vi "ECT verification.vi"(0 ".NET Refnum in":refnum<k24>, 5 "Cal ECT (sec)":u16, 7 "Time remaining (sec)":u16, 11 "error in":errorcluster) -> (3 "Expected SSD":string, 4 ".NET Refnum out":refnum<k24>, 6 "Expected ECT (sec)":u16, 8 "Actual ECT (sec)":u16, 10 "ECT Pass/Fail":bool, 14 "Report Text":string, 15 "error out":errorcluster)   [LabVIEW 2016, in "TL27.lvlib"]
uses:
  Projects/TL27.lvlib
  C:/Automation/DLLs/PC Dot Net/GeaCommunication.dll
  Common/LabVIEW GEA2 Toolkit/LabVIEW_GEA2_Toolkit.lvlibp/type defs/Source_Destination.ctl
  Common/LabVIEW GEA2 Toolkit/LabVIEW_GEA2_Toolkit.lvlibp/type defs/ERD Read Data In.ctl
  Common/LabVIEW GEA2 Toolkit/LabVIEW_GEA2_Toolkit.lvlibp/type defs/Data Type.ctl
  Valew Common/Display/controls/HEUI_Display_Care.ctl
  Valew Common/Display/controls/HEUI_Display.ctl
  Valew Common/Display/controls/Cycle Selection Enum.ctl
  Valew Common/Display/controls/Stain Enum.ctl
  Valew Common/Display/controls/Temp Enum.ctl
  Valew Common/Display/controls/Soil Enum.ctl
  Valew Common/Display/controls/Spin Enum.ctl
  Valew Common/Display/controls/750 Status Enum.ctl
  Common/LabVIEW GEA2 Toolkit/LabVIEW_GEA2_Toolkit.lvlibp
panel:
  out "Diffrence":i16
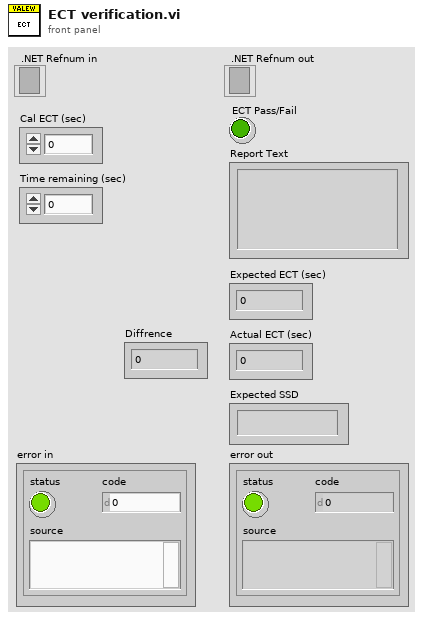
[diagram p1: front panel]
types:
  T1 = typedef "LabVIEW_GEA2_Toolkit.lvlibp/Source_Destination.ctl" = cluster{"Source":u8, "Destination":u8}
  T2 = typedef "LabVIEW_GEA2_Toolkit.lvlibp/ERD Read Data In.ctl" = cluster{"ERD Number":u16, "Data Type":T3}
  T3 = typedef "LabVIEW_GEA2_Toolkit.lvlibp/Data Type.ctl" = enum16{"string", "boolean", "uint8_t", "uint16_t", "uint32_t", "uint64_t", "int8_t", "int16_t", "int32_t", "int64_t"}
  T4 = typedef "TL27.lvlib/HEUI_Display.ctl" = cluster{"SSD":string, "Cycle Selection":T5, "Stain Selection":T6, "Temp Level":T7, "Soil Level":T8, "Spin Level":T9, "750 Status":T10, "Start":bool, "Pause/WiFi":bool, "Lock Controls":bool, "Lid Lock":bool, "Extra Rinse":bool, "Deep Rinse":bool, "Auto Soak":bool, "Warm Rinse":bool, "Deep Fill":bool, "My Cycle":bool, "Delay Wash":bool, "Spin Stop":bool, "Delay":bool, "Fill":bool, "Soak":bool, "Wash":bool, "Rinse":bool, "Spin":bool}
  T5 = typedef "TL27.lvlib/Cycle Selection Enum.ctl" = enum16{"Colors", "Easy Care", "Delicates", "Hand Wash", "Active Wear", "Speed Wash", "Rinse and Spin", "Drain and Spin", "Basket Clean", "Jeans", "Heavy Duty", "Bulky Items", "Towels", "Whites", "Off", "*Incorrect*"}
  T6 = typedef "TL27.lvlib/Stain Enum.ctl" = enum16{"Tomato", "Wine", "Blood", "Grass", "Dirt", "Off", "*Incorrect*"}
  T7 = typedef "TL27.lvlib/Temp Enum.ctl" = enum16{"Hot", "Warm", "Colors", "Cool", "Cold", "Tap Cold", "Off", "*Incorrect*"}
  T8 = typedef "TL27.lvlib/Soil Enum.ctl" = enum16{"Extra Heavy", "Heavy", "Normal", "Light", "Off", "*Incorrect*"}
  T9 = typedef "TL27.lvlib/Spin Enum.ctl" = enum16{"Max Spin", "More Spin", "Normal Spin", "No Spin", "Off", "*Incorrect*"}
  T10 = typedef "TL27.lvlib/750 Status Enum.ctl" = enum16{"Fill", "Wash", "Rinse", "Spin", "Off", "*Incorrect*"}
  T11 = typedef "TL27.lvlib/HEUI_Display_Care.ctl" = cluster{"SSD":bool, "Cycle Selection":bool, "Stain Selection":bool, "Temp Level":bool, "Soil Level":bool, "Spin Level":bool, "750 Status":bool, "Start":bool, "Pause/WiFi":bool, "Lock Controls":bool, "Lid Lock":bool, "Extra Rinse":bool, "Deep Rinse":bool, "Auto Soak":bool, "Warm Rinse":bool, "Deep Fill":bool, "My Cycle":bool, "Delay Wash":bool, "Spin Stop":bool, "Delay":bool, "Fill":bool, "Soak":bool, "Wash":bool, "Rinse":bool, "Spin":bool}
  T12 = typedef "LabVIEW_GEA2_Toolkit.lvlibp/ERD Read Data Out.ctl" = cluster{"ERD Number":u16, "Data":string}
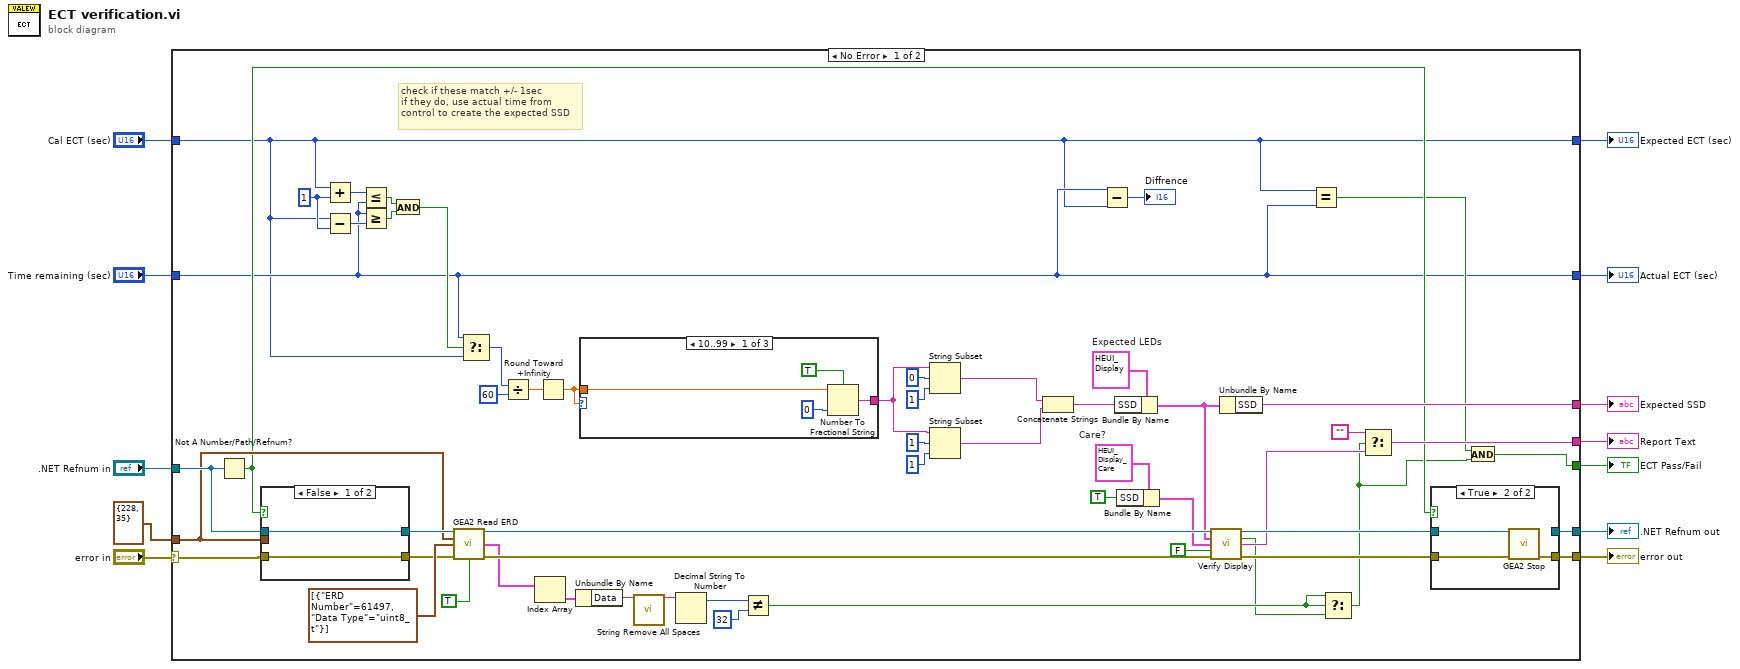
[diagram p0: block diagram]
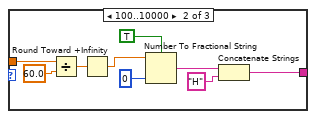
[diagram p2: hidden frame]
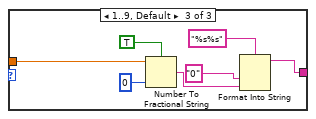
[diagram p3: hidden frame]
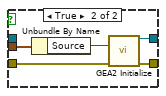
[diagram p5: hidden frame]
diagram:
  n1 = case shown="No Error" "error in" {
    selector: "error in" -> [w40 w102]
    tunnel: [w35 w102] -> w12
    tunnel: [w36 w103] -> w11
    tunnel: [w52 _] -> w10
    tunnel: [w18 _] -> w9
    tunnel: ".NET Refnum in" -> [w51 w103]
    tunnel: "Time remaining (sec)" -> [w17 w101]
    tunnel: "Cal ECT (sec)" -> [w15 _]
    tunnel: [w15 _] -> w6
    tunnel: [w48 _] -> w5
    tunnel: T1 {"Source"=228, "Destination"=35} ("GEA Inputs") -> [w41 _]
    tunnel: [w17 w101] -> w2
    frame No Error {
      w31 = u16 1 ("y")
      w62 = T4 {"SSD"="", "Cycle Selection"=enum."Colors", "Stain Selection"=enum."Tomato", "Temp Level"=enum."Hot", "Soil Level"=enum."Extra Heavy", "Spin Level"=enum."Max Spin", "750 Status"=enum."Fill", "Start"=FALSE, "Pause/WiFi"=FALSE, "Lock Controls"=FALSE, "Lid Lock"=FALSE, "Extra Rinse"=FALSE, "Deep Rinse"=FALSE, "Auto Soak"=FALSE, "Warm Rinse"=FALSE, "Deep Fill"=FALSE, "My Cycle"=FALSE, "Delay Wash"=FALSE, "Spin Stop"=FALSE, "Delay"=FALSE, "Fill"=FALSE, "Soak"=FALSE, "Wash"=FALSE, "Rinse"=FALSE, "Spin"=FALSE}  # Expected LEDs
      w63 = T11 {"SSD"=FALSE, "Cycle Selection"=FALSE, "Stain Selection"=FALSE, "Temp Level"=FALSE, "Soil Level"=FALSE, "Spin Level"=FALSE, "750 Status"=FALSE, "Start"=FALSE, "Pause/WiFi"=FALSE, "Lock Controls"=FALSE, "Lid Lock"=FALSE, "Extra Rinse"=FALSE, "Deep Rinse"=FALSE, "Auto Soak"=FALSE, "Warm Rinse"=FALSE, "Deep Fill"=FALSE, "My Cycle"=FALSE, "Delay Wash"=FALSE, "Spin Stop"=FALSE, "Delay"=FALSE, "Fill"=FALSE, "Soak"=FALSE, "Wash"=FALSE, "Rinse"=FALSE, "Spin"=FALSE}  # Care?
      # "check if these match +/- 1sec\nif they do, use actual time from\ncontrol to create the expected SSD"
      n2 = Not A Number/Path/Refnum?(number/path/refnum=w51) -> (NaN/Path/Refnum?=w37:bool)
      n3 = case shown="False" w37 {
        tunnel: [w94 w100] -> w49
        tunnel: w40 -> [w94 w99]
        tunnel: [w95 w98] -> w50
        tunnel: w51 -> [w95 _]
        tunnel: w41 -> [_ w97]
        frame False {
        }
        frame True {
          n4 = Unbundle By Name(w97) -> ("Source"=w96:u8)
          n5 = call "GEA2 Initialize.vi"("Source Address"=w96, "error in"=w99) -> ("GEA2 Reference Out"=w98:refnum<k24>, "error out"=w100:errorcluster)  [unwired: 11 in, 1 out]
        }
      }
      n6 = Add(x=w15, y=w31) -> (x+y=w30:u16)
      n7 = Subtract(x=w15, y=w31) -> (x-y=w25:u16)
      n8 = Less Or Equal?(x=w30, y=w17) -> (x <= y?=w28:bool)
      n9 = Greater Or Equal?(x=w17, y=w25) -> (x >= y?=w29:bool)
      n10 = And(x=w28, y=w29) -> (x .and. y?=w27:bool)
      n11 = call "GEA2 Read ERD.vi"("GEA2 Reference In"=w50, "GEA Inputs"=w41, "Read ERD List"=T2[] [{"ERD Number"=61497, "Data Type"=enum."uint8_t"}], "Error In"=w49, "Verify ERD Response?"=TRUE) -> ("GEA2 Reference Out"=w67:refnum<k24>, "ERD Data Out"=w65:T12[], "Error Out"=w68:errorcluster)  [unwired: 7 in, 1 out]
      n12 = Select(t=w17, s=w27, f=w15) -> (s? t:f=w26:u16)
      n13 = Divide(x=w26, y=60) -> (x/y=w61:dbl)
      n14 = Index Array(array=w65) -> (element=w23:T12)  [unwired: 1 in]
      n15 = Round Toward +Infinity(x=w61) -> (ceil(x): smallest int >= x=w66:dbl)
      n16 = Unbundle By Name(w23) -> ("Data"=w57:string)
      n17 = case shown="10..99" w66 {
        tunnel: [w70 w73 w84] -> w43
        tunnel: w66 -> [w69 w74 w83]
        frame 10..99 {
          n18 = Number To Fractional String(use system decimal point (T)=TRUE, number=w69, precision (6)=i16 0) -> (F-format string=w70:string)  [unwired: 1 in]
        }
        frame 100..10000 {
          n19 = Divide(x=w74, y=60.0) -> (x/y=w78:dbl)
          n20 = Round Toward +Infinity(x=w78) -> (ceil(x): smallest int >= x=w77:dbl)
          n21 = Number To Fractional String(use system decimal point (T)=TRUE, number=w77, precision (6)=i16 0) -> (F-format string=w76:string)  [unwired: 1 in]
          n22 = Concatenate Strings(w76, "H") -> (w73:string)
        }
        frame 1..9, Default {
          n23 = Number To Fractional String(use system decimal point (T)=TRUE, number=w83, precision (6)=i16 0) -> (F-format string=w88:string)  [unwired: 1 in]
          n24 = Format Into String(format string="%s%s", "0" ("input 1"), w88) -> (resulting string=w84:string)  [unwired: 2 in, 1 out]
        }
      }
      n25 = call "String Remove All Spaces.vi"("Input String"=w57) -> ("Spaces Removed"=w56:string)  [unwired: 13 in, 1 out]
      n26 = Decimal String To Number(string=w56) -> (offset past number=w55:i32)  [unwired: 2 in, 1 out]
      n27 = Not Equal?(x=w55, y=32) -> (x != y?=w22:bool)
      n28 = String Subset(string=w43, offset (0)=0, length (rest)=1 ("length (rest)")) -> (substring=w14:string)
      n29 = String Subset(string=w43, offset (0)=1, length (rest)=1 ("length (rest)")) -> (substring=w13:string)
      n30 = Concatenate Strings(w14, w13) -> (w42:string)
      n31 = Subtract(x=w17, y=w15) -> (x-y=→"Diffrence":u16)
      n32 = Bundle By Name(cluster=w62, "SSD"=w42) -> (w34:T4)
      n33 = Bundle By Name(cluster=w63, "SSD"=TRUE) -> (w33:T11)
      n34 = call "Verify Display.vi"("GEA2 Reference In"=w67, "Expected LEDs"=w34, "Care?"=w33, "Ignore Brightness?"=FALSE, "Error In"=w68) -> ("GEA2 Reference Out"=w39:refnum<k24>, "Pass/Fail?"=w21:bool, "Report Text"=w24:string, "Error Out"=w38:errorcluster)  [unwired: 7 in]
      n35 = Unbundle By Name(w34) -> ("SSD"=w48:string)
      n36 = Equal?(x=w15, y=w17) -> (x = y?=w20:bool)
      n37 = Select(t=w22, s=w22, f=w21) -> (s? t:f=w19:bool)
      n38 = Select(t="", s=w19, f=w24) -> (s? t:f=w52:string)
      n39 = case shown="True" w37 {
        tunnel: [w90 w93] -> w35
        tunnel: w39 -> [w89 w92]
        tunnel: w38 -> [w90 w91]
        tunnel: [w89 _] -> w36
        frame False {
        }
        frame True {
          n40 = call "GEA2 Stop.vi"("GEA2 Reference In"=w92, "Error In"=w91) -> ("Error Out"=w93:errorcluster)  [unwired: 13 in]
        }
      }
      n41 = And(x=w20, y=w19) -> (x .and. y?=w18:bool)
    }
    frame Error {
    }
  }
  "Expected SSD" <- w5
  "Actual ECT (sec)" <- w2
  "ECT Pass/Fail" <- w9
  "error out" <- w12
  ".NET Refnum out" <- w11
  "Report Text" <- w10
  "Expected ECT (sec)" <- w6
